vi "Create Two Column Table HTML From Channel List.vi"(6 "Instance ID":string, 7 "engine configuration in":refnum<class "engine configuration.lvclass">, 8 "Node#":i32, 9 "Color":string="invis", 10 "Title":string, 11 "Channels":refnum<class "TBM channel.lvclass">[](array[class])) -> (2 "Table HTML":string, 3 "Channel and Node Pairs":T1[](array[typedef]))   [LabVIEW 2013]
uses:
  <vilib>/NI/Tag Bus Module Framework/channel/TBM channel.lvclass
  Channel to Port Pair.ctl
  <vilib>/NI/Module Execution Interface/Engine Configuration/engine configuration.lvclass
  <vilib>/NI/Tag Bus Module Framework/channel/channel classification.ctl
  <vilib>/NI/Tag Bus/tag/tag descriptor.lvclass/tag descriptor.ctl
  <vilib>/NI/Tag Bus/tag/read tag name.vi
  <vilib>/NI/Tag Bus/tag/tag descriptor.lvclass
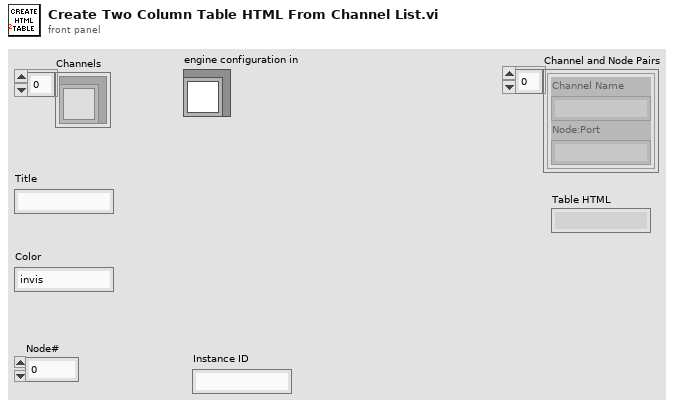
[diagram p1: front panel]
types:
  T1 = typedef "Channel to Port Pair.ctl" = cluster{"Channel Name":string, "Node:Port":string}
  T2 = typedef "TBM channel.lvclass/channel classification.ctl" = enum16{"input data", "output data", "processing parameter", "processing result"}
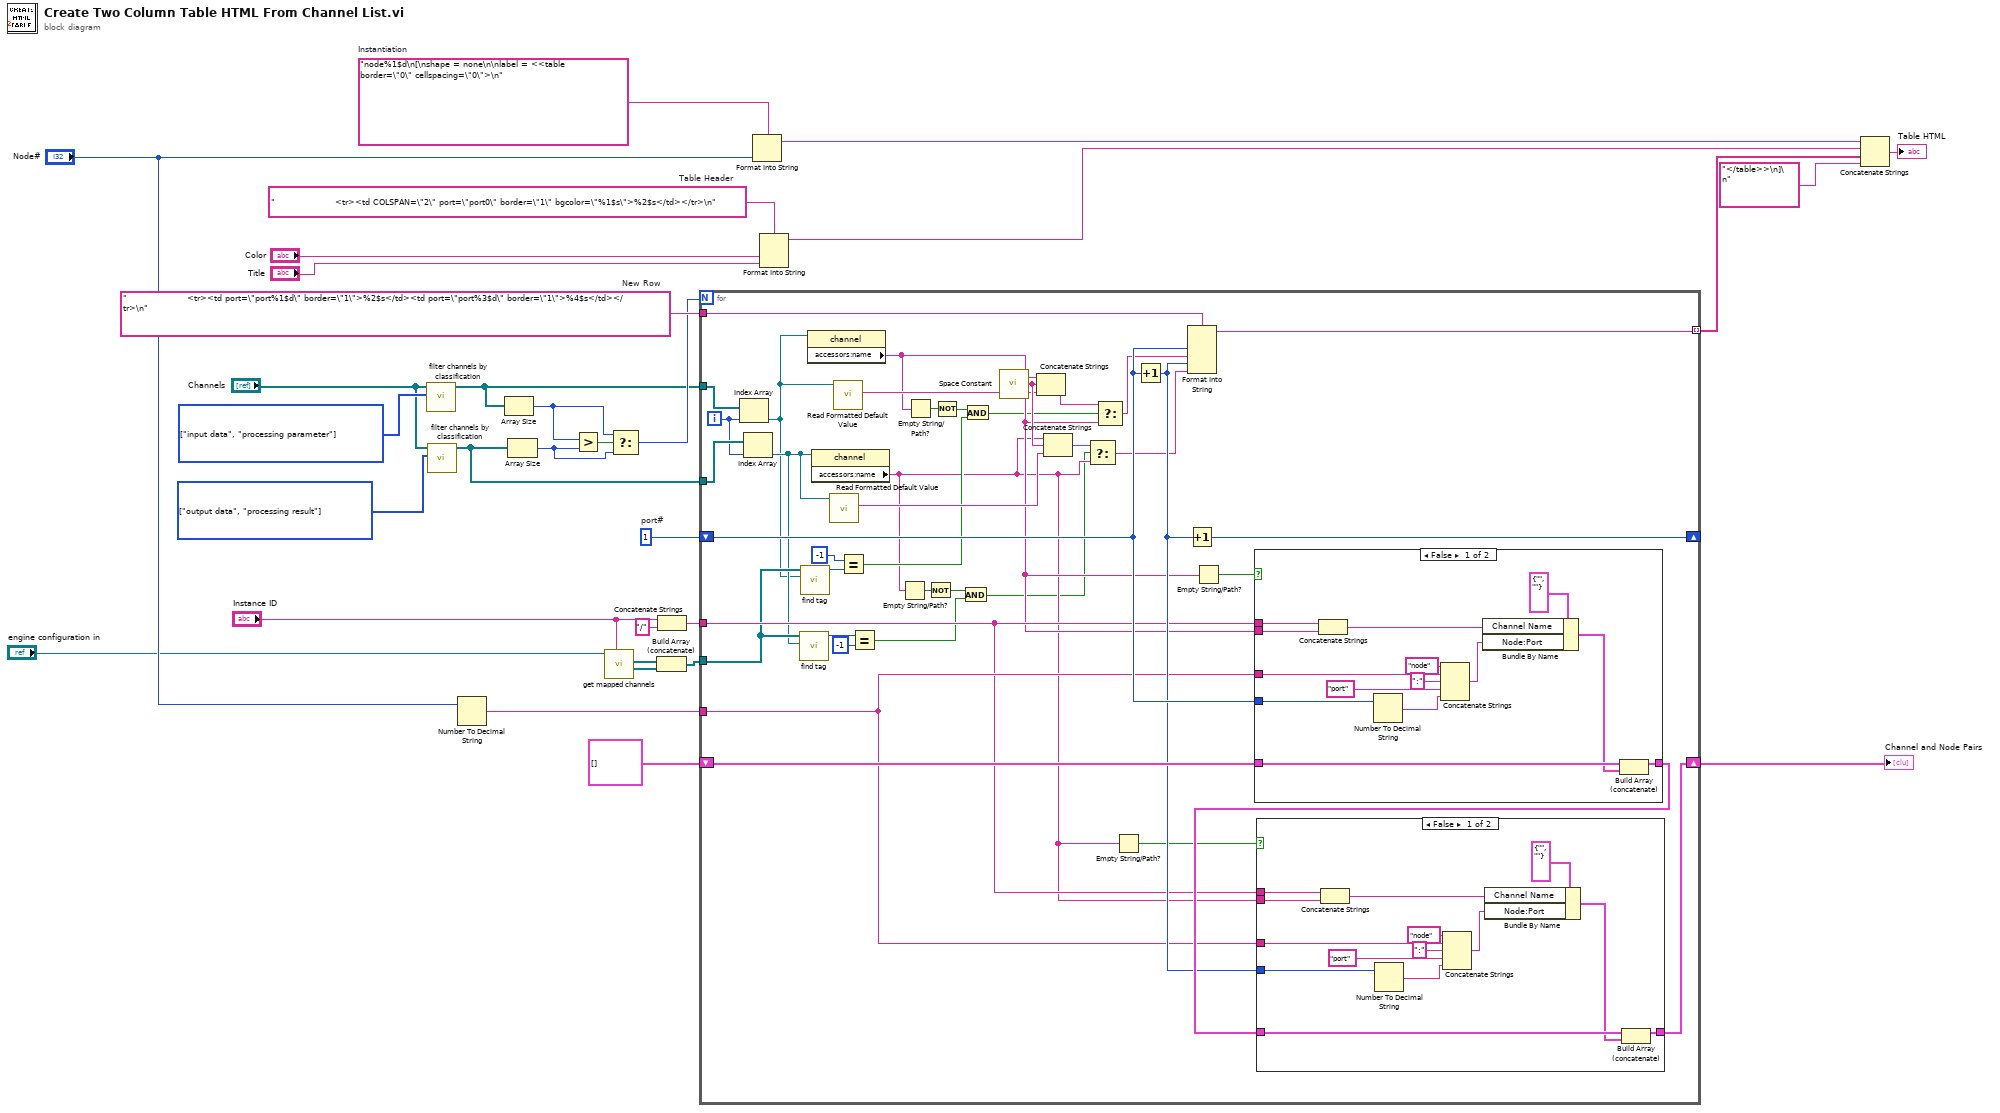
[diagram p0: block diagram]
diagram:
  w12 = 1  # port#
  w19 = T2[] [enum."output data", enum."processing result"] items=["input data", "output data", "processing parameter", "processing result"] ("allowed classifications")
  w21 = T2[] [enum."input data", enum."processing parameter"] items=["input data", "output data", "processing parameter", "processing result"] ("allowed classifications")
  w24 = "node%1$d\n[\nshape = none\n\nlabel = <<table border=\"0\" cellspacing=\"0\">\n"  # Instantiation
  w29 = "                    <tr><td COLSPAN=\"2\" port=\"port0\" border=\"1\" bgcolor=\"%1$s\">%2$s</td></tr>\n"  # Table Header
  w31 = "                    <tr><td port=\"port%1$d\" border=\"1\">%2$s</td><td port=\"port%3$d\" border=\"1\">%4$s</td></tr>\n"  # New Row
  n1 = call <vilib>:"filter channels by classification.vi"("allowed classifications"=w21, "channels in"="Channels") -> ("channels out"=w13:refnum<class "TBM channel.lvclass">[])  [unwired: 9 in]
  n2 = call <vilib>:"filter channels by classification.vi"("allowed classifications"=w19, "channels in"="Channels") -> ("channels out"=w14:refnum<class "TBM channel.lvclass">[])  [unwired: 9 in]
  n3 = Number To Decimal String(number="Node#") -> (decimal integer string=w8:string)  [unwired: 1 in]
  n4 = Array Size(array=w13) -> (size(s)=w17:i32)
  n5 = Array Size(array=w14) -> (size(s)=w16:i32)
  n6 = Greater?(x=w17, y=w16) -> (0:w18:bool)
  n7 = call <vilib>:"get mapped channels.vi"("owner"="Instance ID", "engine configuration in"="engine configuration in") -> ("write channels"=w2:refnum<class "TBM channel.lvclass">[], "read channels"=w3:refnum<class "TBM channel.lvclass">[])  [unwired: 5 in, 3 out]
  n8 = Select(t=w17, s=w18, f=w16) -> (s? t:f=w15:i32)
  n9 = Build Array (concatenate)(w3, w2) -> (w1:refnum<class "TBM channel.lvclass">[])
  n10 = Concatenate Strings("Instance ID", "/" ("string")) -> (w5:string)
  n11 = for {
    N: w15 -> [_]
    tunnel: [w70] -> w25 mode=indexing
    tunnel: w31 -> [w69]
    tunnel: w14 -> [w67]
    tunnel: w13 -> [w68]
    shift-right: [w66] -> _
    shift-left: w12 -> [w63]
    shift-right: [w61] -> w7
    shift-left: T1[] [] ("Channel and Node Pairs") -> [w64]
    tunnel: w5 -> [w55]
    tunnel: w8 -> [w59]
    tunnel: w1 -> [w46]
    i -> [w56]
    n12 = Index Array(array=w68, index=w56) -> (element=w43:refnum<class "TBM channel.lvclass">)
    n13 = Index Array(array=w67, index=w56) -> (element=w45:refnum<class "TBM channel.lvclass">)
    n14 = call <vilib>:"find tag.vi"("tag"=w45, "tags in"=w46) -> ("index"=w48:i32)  [unwired: 9 in]
    n15 = call <vilib>:"find tag.vi"("tag"=w43, "tags in"=w46) -> ("index"=w53:i32)  [unwired: 9 in]
    n16 = property class="channel"(reference=w43) -> ("accessors:name"=w41:string)  [unwired: 1 in, 2 out]
    n17 = property class="channel"(reference=w45) -> ("accessors:name"=w35:string)  [unwired: 1 in, 2 out]
    n18 = call "Read Formatted Default Value.vi"("channel"=w45) -> ("Formatted Default"=w44:string)  [unwired: 9 in, 1 out]
    n19 = call "Read Formatted Default Value.vi"("channel"=w43) -> ("Formatted Default"=w42:string)  [unwired: 9 in, 1 out]
    n20 = Equal?(x=-1, y=w53) -> (x = y?=w38:bool)
    n21 = Equal?(x=w48, y=-1) -> (x = y?=w33:bool)
    n22 = Empty String/Path?(string/path=w35) -> (empty?=w36:bool)
    n23 = Empty String/Path?(string/path=w41) -> (empty?=w40:bool)
    n24 = Not(x=w36) -> (.not. x?=w34:bool)
    n25 = Not(x=w40) -> (.not. x?=w39:bool)
    n26 = And(x=w34, y=w33) -> (x .and. y?=w32:bool)
    n27 = And(x=w39, y=w38) -> (x .and. y?=w37:bool)
    n28 = call <vilib>:"Space Constant.vi"() -> ("String"=w50:string)
    n29 = Concatenate Strings(w41, w50, w42) -> (w57:string)
    n30 = Concatenate Strings(w35, w50, w44) -> (w51:string)
    n31 = Select(t=w51, s=w32, f=w35) -> (s? t:f=w49:string)
    n32 = Select(t=w57, s=w37, f=w41) -> (s? t:f=w52:string)
    n33 = Empty String/Path?(string/path=w35) -> (empty?=w58:bool)
    n34 = Increment(x=w63) -> (x+1=w60:i32)
    n35 = Format Into String(format string=w69, w63, w52, w60, w49) -> (resulting string=w70:string)  [unwired: 2 in, 1 out]
    n36 = Increment(x=w60) -> (x+1=w66:i32)
    n37 = Empty String/Path?(string/path=w41) -> (empty?=w65:bool)
    n38 = case shown="False" w65 {
      tunnel: w41 -> [w97 _]
      tunnel: w55 -> [w98 _]
      tunnel: w64 -> [w95 w100]
      tunnel: [w93 w100] -> w62
      tunnel: w59 -> [w88 _]
      tunnel: w63 -> [w87 _]
      frame False {
        n39 = Concatenate Strings(w98, w97) -> (w96:string)
        n40 = Number To Decimal String(number=w87) -> (decimal integer string=w89:string)  [unwired: 1 in]
        n41 = Concatenate Strings("node" ("string"), w88, ":" ("string"), "port" ("string"), w89) -> (w86:string)
        n42 = Bundle By Name(cluster=T1 {"Channel Name"="", "Node:Port"=""} ("Channel to Port Pair"), "Channel Name"=w96, "Node:Port"=w86) -> (w94:T1)
        n43 = Build Array (concatenate)(w95, w94) -> (w93:T1[])
      }
      frame True {
      }
    }
    n44 = case shown="False" w58 {
      tunnel: w35 -> [w82 _]
      tunnel: w55 -> [w83 _]
      tunnel: w62 -> [w80 w85]
      tunnel: [w78 w85] -> w61
      tunnel: w59 -> [w73 _]
      tunnel: w60 -> [w72 _]
      frame False {
        n45 = Concatenate Strings(w83, w82) -> (w81:string)
        n46 = Number To Decimal String(number=w72) -> (decimal integer string=w74:string)  [unwired: 1 in]
        n47 = Concatenate Strings("node" ("string"), w73, ":" ("string"), "port" ("string"), w74) -> (w71:string)
        n48 = Bundle By Name(cluster=T1 {"Channel Name"="", "Node:Port"=""} ("Channel to Port Pair"), "Channel Name"=w81, "Node:Port"=w71) -> (w79:T1)
        n49 = Build Array (concatenate)(w80, w79) -> (w78:T1[])
      }
      frame True {
      }
    }
  }
  "Channel and Node Pairs" <- w7
  n50 = Format Into String(format string=w24, "Node#") -> (resulting string=w23:string)  [unwired: 2 in, 1 out]
  n51 = Format Into String(format string=w29, "Color", "Title") -> (resulting string=w26:string)  [unwired: 2 in, 1 out]
  n52 = Concatenate Strings(w23, w26, w25, "</table>>\n]\n") -> (→"Table HTML":string)
